vi "Read_OTParametersSP.vi"() -> ()   [LabVIEW 2016]
uses:
  <vilib>/NI/Current Value Table/DataTypes/U16_Read.vi
  <vilib>/NI/Current Value Table/Type to Enum.vi
  <vilib>/NI/Current Value Table/DataTypes/U16_Type To Enum.vi
  <vilib>/Utility/file.llb/Read Delimited Spreadsheet (string).vi
  <vilib>/NI/Current Value Table/FGVs/CVT Globals.vi
  <vilib>/NI/Current Value Table/FGVs/Tag Memory.vi
  <vilib>/NI/Current Value Table/Memory Block.vi
  <vilib>/NI/Current Value Table/DataTypes/U16_Memory Block.vi
  <vilib>/NI/Current Value Table/Current Value Table.lvlib
panel:
  in  "Cancel Button":bool
  out "?":cluster{u16}[](array[cluster])
  out "?":cluster{u16}[](array[cluster])
  out "?":cluster{u16}[](array[cluster])
  out "?":cluster{u16}[](array[cluster])
  out "?":cluster{u16}[](array[cluster])
  out "?":cluster{u16}[](array[cluster])
  # "O.T Parameters S.P"
  # "O2 Gas Pressure"
  # "Bar"
  # "N2 Gas Pressure 1"
  # "Bar"
  # "Velocity"
  # "ft/m"
  # "N2 Gas Pressure 2"
  # "Bar"
  # "Room Temperature"
  # "Degree C"
  # "Relative Humidity"
  # "%"
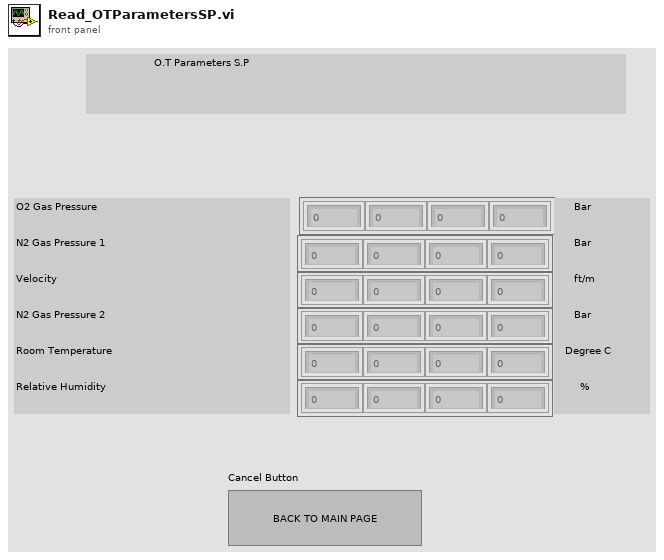
[diagram p1: front panel]
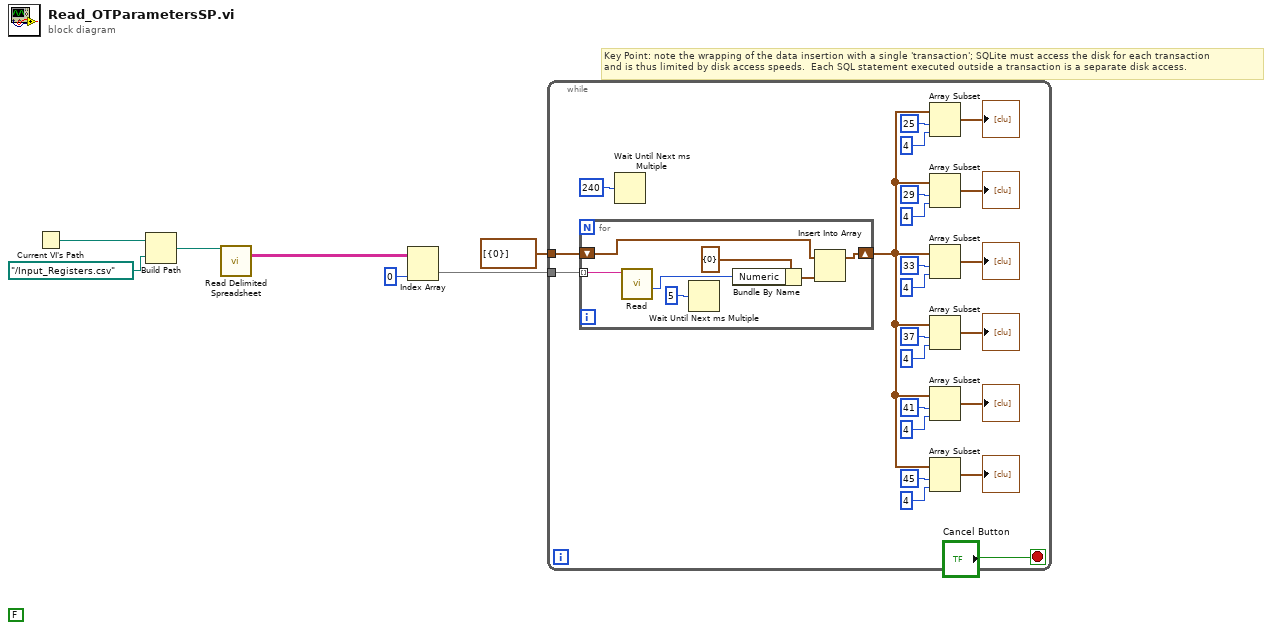
[diagram p0: block diagram]
diagram:
  (unwired) FALSE
  # "Key Point: note the wrapping of the data insertion with a single 'transaction'; SQLite must access the disk for each transaction\nand is thus limited by disk access speeds.  Each SQL statement executed outside a transaction is a separate disk access."
  n1 = Current VI's Path() -> (path=w3:path)
  n2 = Build Path(base path=w3, name or relative path=path "../Input_Registers.csv") -> (appended path=w1:path)
  n3 = call-poly <vilib>:"Read Delimited Spreadsheet.vi"("file path (dialog if empty)"=w1) -> ("all rows"=w6:string[][])  [unwired: 9 in, 5 out]
  n4 = Index Array "Index Array"(array=w6, index (col)=0 ("disabled index (col)")) -> (element=w4:string[])  [unwired: 1 in]
  n5 = while {
    tunnel: cluster{"Numeric":u16}[] [{"Numeric"=0}] ("output array") -> [w30]
    tunnel: w4 -> [w29]
    stop <- "Cancel Button" stop-if-true
    n6 = for {
      shift-right: [w34] -> w19
      shift-left: w30 -> [w35]
      tunnel: w29 -> [w33] mode=indexing
      n7 = call-poly <vilib>:"Read.vi"("Tag Name"=w33) -> ("Value"=w32:u16)  [unwired: 9 in, 1 out]
      n8 = Wait Until Next ms Multiple(millisecond multiple=u32 5 ("millisecond timer value")) -> ()  [unwired: 1 out]
      n9 = Bundle By Name(cluster=cluster{"Numeric":u16} {"Numeric"=0} ("Cluster"), "Numeric"=w32) -> (w36:cluster{"Numeric":u16})
      n10 = Insert Into Array(array=w35, new element=w36) -> (w34:cluster{"Numeric":u16}[])  [unwired: 1 in]
    }
    n11 = Wait Until Next ms Multiple(millisecond multiple=u32 240 ("milliseconds to wait")) -> ()  [unwired: 1 out]
    n12 = Array Subset(array=w19, index=25, length=4) -> (→"?":cluster{"Numeric":u16}[])
    n13 = Array Subset(array=w19, index=29, length=4) -> (→"?":cluster{"Numeric":u16}[])
    n14 = Array Subset(array=w19, index=33, length=4) -> (→"?":cluster{"Numeric":u16}[])
    n15 = Array Subset(array=w19, index=37, length=4) -> (→"?":cluster{"Numeric":u16}[])
    n16 = Array Subset(array=w19, index=41, length=4) -> (→"?":cluster{"Numeric":u16}[])
    n17 = Array Subset(array=w19, index=45, length=4) -> (→"?":cluster{"Numeric":u16}[])
  }
